vi "Load config.vi"(8 "error in (no error)":errorcluster) -> (0 "error out":errorcluster, 3 "Datos Adquisición out":T1={"Equipo a Utilizar"=enum."TDS 2012B Osciloscope", "Montura"=enum."Motor Bipolar", "Datos Zaber"={"Sentido de Adquisición"=FALSE, "Comenzar Desde Home?"=FALSE, "Distancia a recorrer (um)"=0.0, "Pasos motor"=0, "Distancia entre Lecturas (um)"=0.0, "Puerto"=""}, "Datos Bipolar/Unipolar"={"Puerto COM"="", "Pasos entre Lecturas"=0, "Numero de lecturas"=0, "Sentido del motor"=TRUE}, "Datos Archivo"={"Ruta Archivo"=path "", "Nombre de Prueba"=""}, "Datos actuales"={"Montura"="", "Equipo"="", "Posición Actual"="", "Distancia Total a recorrer"="", "distancia Entre lecturas"="", "Pasos entre lecturas"=""}, "Datos a Guardar In"={"Datos Cursor Tektronix"="", "Datos Lokin"="", "Posición Cero"=0.0, "Posición Actual"=0.0}, "Datos Osciloscopio"={"Sesión Visa Osciloscopio"="Tektronix_TDS2012C", "Tipo de Adquisición"=enum."Voltaje Pico Pico", "Canal a Utilizar"=enum."Canal 1", "Parametros de Adquisición"=enum."Una Muestra", "Número Promedio"=2}, "Datos Lock In"={"Visa Lock in"="Tektronix_TDS2012C"}} {"Datos Osciloscopio"."Número Promedio" min=2 max=20; "Datos a Guardar In"."Posición Actual" format="%#_10f"; "Datos a Guardar In"."Posición Cero" format="%#_10f"; "Datos Bipolar/Unipolar"."Numero de lecturas" max=910098 step=1})   [LabVIEW 2020]
uses:
  <vilib>/Utility/config.llb/NI_LVConfig.lvlib
  <vilib>/Utility/config.llb/Read Key (U32).vi
  H:/Mi unidad/Departamento de Ingenieria/Investigadores/Gabriel Ramos/Proyecto Monturas v13/LV Source/Type Definitions/Tipos de montura.ctl
  Type Definitions/Datos Zaber.ctl
  Type Definitions/parametros motores.ctl
  Type Definitions/Datos a Guardar.ctl
  Type Definitions/datos osciloscopio.ctl
  Type Definitions/Asistente de adquisicion Cluster.ctl
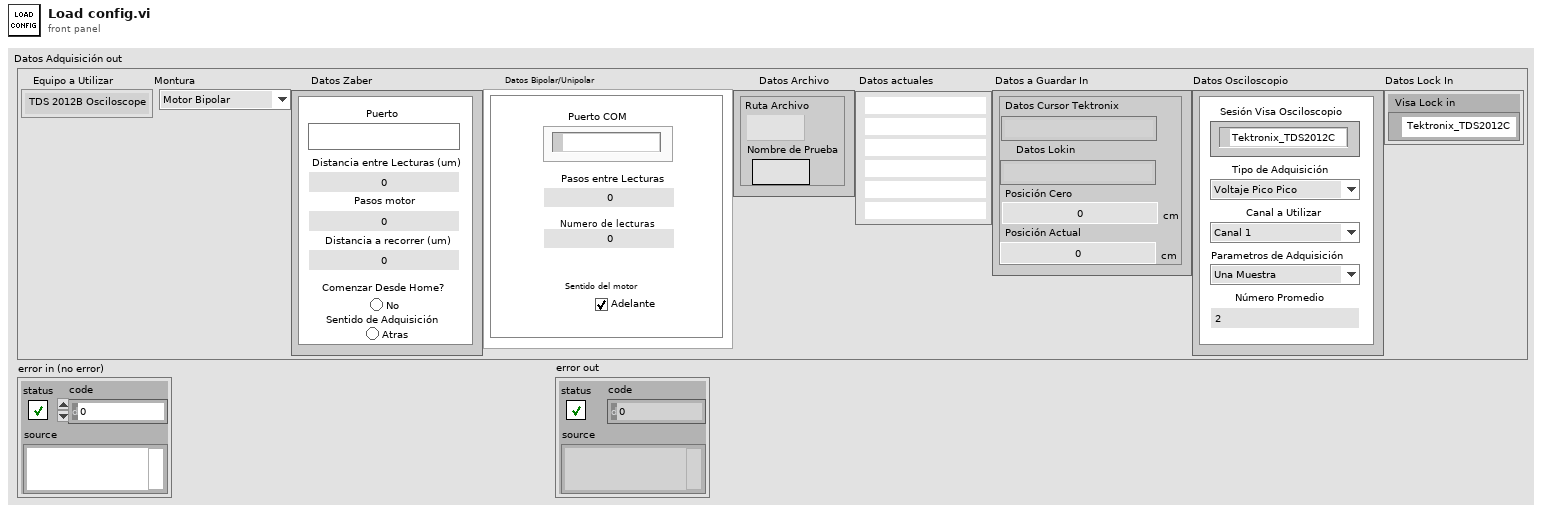
[diagram p1: front panel]
types:
  T1 = typedef "Asistente de adquisicion Cluster.ctl" = cluster{"Equipo a Utilizar":enum16{"SR830 Lock In", "TDS 2012B Osciloscope"}, "Montura":T2, "Datos Zaber":T3, "Datos Bipolar/Unipolar":T4, "Datos Archivo":cluster{"Ruta Archivo":path, "Nombre de Prueba":string}, "Datos actuales":cluster{"Montura":string, "Equipo":string, "Posición Actual":string, "Distancia Total a recorrer":string, "distancia Entre lecturas":string, "Pasos entre lecturas":string}, "Datos a Guardar In":T5, "Datos Osciloscopio":T6, "Datos Lock In":cluster{"Visa Lock in":refnum<visa-resource-name>}}
  T2 = typedef "Tipos de montura.ctl" = enum16{"Zaber T-LSR450B", "Zaber-T-LSR300B", "Zaber-T-LSRxxx", "Motor Bipolar", "Motor Unipolar"}
  T3 = typedef "Datos Zaber.ctl" = cluster{"Sentido de Adquisición":bool, "Comenzar Desde Home?":bool, "Distancia a recorrer (um)":dbl, "Pasos motor":i32, "Distancia entre Lecturas (um)":dbl, "Puerto":refnum<visa-resource-name>}
  T4 = typedef "parametros motores.ctl" = cluster{"Puerto COM":refnum<visa-resource-name>, "Pasos entre Lecturas":u16, "Numero de lecturas":u32, "Sentido del motor":bool}
  T5 = typedef "Datos a Guardar.ctl" = cluster{"Datos Cursor Tektronix":string, "Datos Lokin":string, "Posición Cero":dbl[unit], "Posición Actual":dbl[unit]}
  T6 = typedef "datos osciloscopio.ctl" = cluster{"Sesión Visa Osciloscopio":refnum<visa-resource-name>, "Tipo de Adquisición":enum16{"Voltaje Pico Pico", "Voltaje RMS", "Cursor Tiempo"}, "Canal a Utilizar":enum16{"Canal 1", "Canal 2", "Canal 1 y 2"}, "Parametros de Adquisición":enum16{"Una Muestra", "Promedio"}, "Número Promedio":i32}
  T7 = typedef "NI_LVConfig.lvlib/Config Data RefNum.ctl" = refnum<k1>
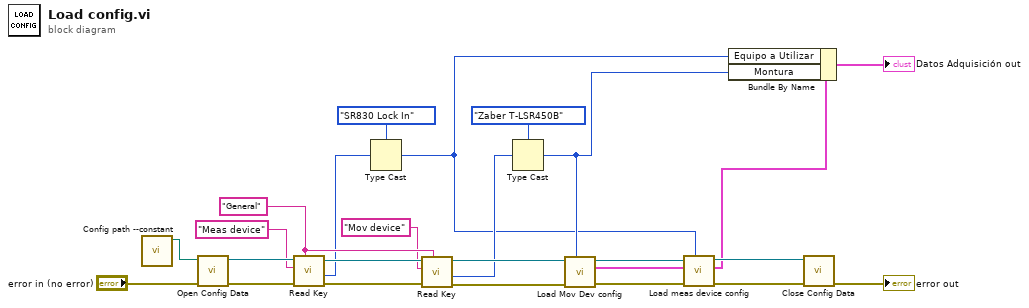
[diagram p0: block diagram]
diagram:
  w15 = "General" ("section")
  n1 = call "Config path --constant.vi"() -> ("appended path"=w23:path)  [unwired: 11 in]
  n2 = call <vilib>:"Open Config Data.vi"("error in (no error)"="error in (no error)", "configuration file path"=w23) -> ("error out"=w24:errorcluster, "refnum"=w21:T7)  [unwired: 7 in, 1 out]
  n3 = call-poly <vilib>:"Read Key.vi"("section"=w15, "error in (no error)"=w24, "key"="Meas device", "refnum"=w21) -> ("error out"=w17:errorcluster, "value"=w4:u32, "refnum out"=w16:T7)  [unwired: 4 in, 1 out]
  n4 = Type Cast(type=enum16{"SR830 Lock In", "TDS 2012B Osciloscope"}."SR830 Lock In" ("Equipo a Utilizar"), x=w4) -> (*(type *) &x=w2:enum16{"SR830 Lock In", "TDS 2012B Osciloscope"})
  n5 = call-poly <vilib>:"Read Key.vi"("section"=w15, "error in (no error)"=w17, "key"="Mov device", "refnum"=w16) -> ("error out"=w12:errorcluster, "value"=w9:u32, "refnum out"=w11:T7)  [unwired: 4 in, 1 out]
  n6 = Type Cast(type=Tipos_de_montura."Zaber T-LSR450B" ("Montura"), x=w9) -> (*(type *) &x=w8:T2)
  n7 = call "Load Mov Dev config.vi"("Montura"=w8, "error in (no error)"=w12, "Refnum in"=w11) -> ("error out"=w10:errorcluster, "Datos Adquisición out"=w3:T1, "refnum out"=w6:T7)  [unwired: 6 in]
  n8 = call "Load meas device config.vi"("Equipo a Utilizar"=w2, "error in (no error)"=w10, "Datos Adquisición"=w3, "Refnum in"=w6) -> ("error out"=w7:errorcluster, "Datos Adquisición out"=w1:T1, "Refnum out"=w5:T7)  [unwired: 5 in]
  n9 = Bundle By Name(cluster=w1, "Equipo a Utilizar"=w2, "Montura"=w8) -> (→"Datos Adquisición out":T1)
  n10 = call <vilib>:"Close Config Data.vi"("error in (no error)"=w7, "refnum"=w5) -> ("error out"=→"error out":errorcluster)  [unwired: 8 in, 1 out]
